vi "PDE_Cal Delta.vi"(9 "# of points":i32, 10 "end":dbl, 11 "start":dbl) -> (3 "delta":dbl)   [LabVIEW 2020, in "NI_PDE.lvlib"]
uses:
  <vilib>/gmath/NI_PDE.lvlib
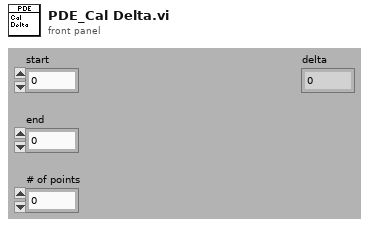
[diagram p1: front panel]
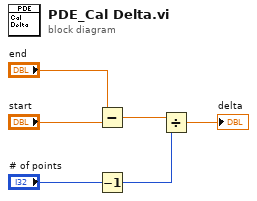
[diagram p0: block diagram]
diagram:
  n1 = Subtract(x="end", y="start") -> (x-y=w3:dbl)
  n2 = Decrement(x="# of points") -> (x-1=w2:i32)
  n3 = Divide(x=w3, y=w2) -> (x/y=→"delta":dbl)
